vi "Address setting.vi"(7 "Address Cluster out输入":T1={"SPU"=refnum, "MPM"=[], "Port_Count"=0.0, "MPM_Count"=0.0, "SPU_Resource"=[], "USB_Resource"=[], "MPM_Communicater"="", "MPM_Count"=0.0, "MPM_Address"=[], "MPM_Portnumber"=[], "SPU_DeviveID"="", "MPM_communcation_method"=[], "TSL_sweepstartwave"=0.0, "TSL_sweepstopwave"=0.0, "TSL_Address"="", "TSL_Communicater"="", "TSL"=refnum, "tsl_communcation_method"=3, "TSL_Portnumber"=0.0} {"tsl_communcation_method" items=["GPIB", "C232C", "TCPIP", "USB"]; "MPM_communcation_method" items=["GPIB", "C232C", "TCPIP", "USB"]}, 8 "错误输入（无错误）":errorcluster caption="error in", 10 "PowerMonitorType":enum16{"DAQ", "MPM_220", "TSL_LOGG"}(ring), 11 "SPU in":refnum<k24>) -> (0 "error out":errorcluster, 1 "Address Cluster out输出":T1={"SPU"=refnum, "MPM"=[], "Port_Count"=0.0, "MPM_Count"=0.0, "SPU_Resource"=[], "USB_Resource"=[], "MPM_Communicater"="", "MPM_Count"=0.0, "MPM_Address"=[], "MPM_Portnumber"=[], "SPU_DeviveID"="", "MPM_communcation_method"=[], "TSL_sweepstartwave"=0.0, "TSL_sweepstopwave"=0.0, "TSL_Address"="", "TSL_Communicater"="", "TSL"=refnum, "tsl_communcation_method"=3, "TSL_Portnumber"=0.0} {"tsl_communcation_method" items=["GPIB", "C232C", "TCPIP", "USB"]; "MPM_communcation_method" items=["GPIB", "C232C", "TCPIP", "USB"]})   [LabVIEW 2017]
doc: "'----Apply to communication parametere from Instrument setting form"
uses:
  CTL/Address Cluster.ctl
  D:/test/ILSTS/LV_IL/LV_IL_Sample_x64/DLL/InstrumentDLL.dll
  DLL/InstrumentDLL.dll
  Share/PowerMonitorType.vi
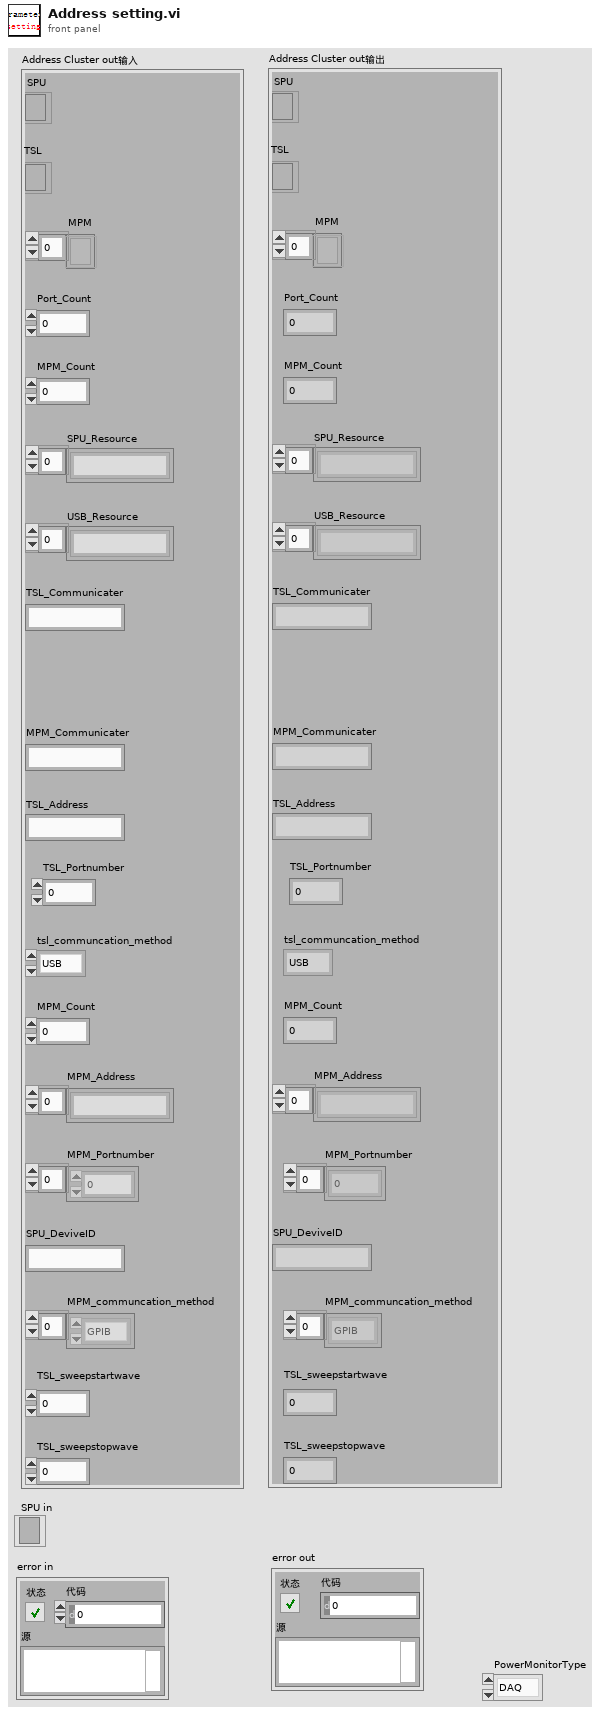
[diagram p1: front panel]
types:
  T1 = typedef "Address Cluster.ctl" = cluster{"SPU":refnum<k24>, "MPM":refnum<k24>[], "Port_Count":dbl, "MPM_Count":dbl, "SPU_Resource":string[], "USB_Resource":string[], "MPM_Communicater":string, "MPM_Count":dbl, "MPM_Address":string[], "MPM_Portnumber":dbl[], "SPU_DeviveID":string, "MPM_communcation_method":i32[], "TSL_sweepstartwave":dbl, "TSL_sweepstopwave":dbl, "TSL_Address":string, "TSL_Communicater":string, "TSL":refnum<k24>, "tsl_communcation_method":i32, "TSL_Portnumber":dbl}
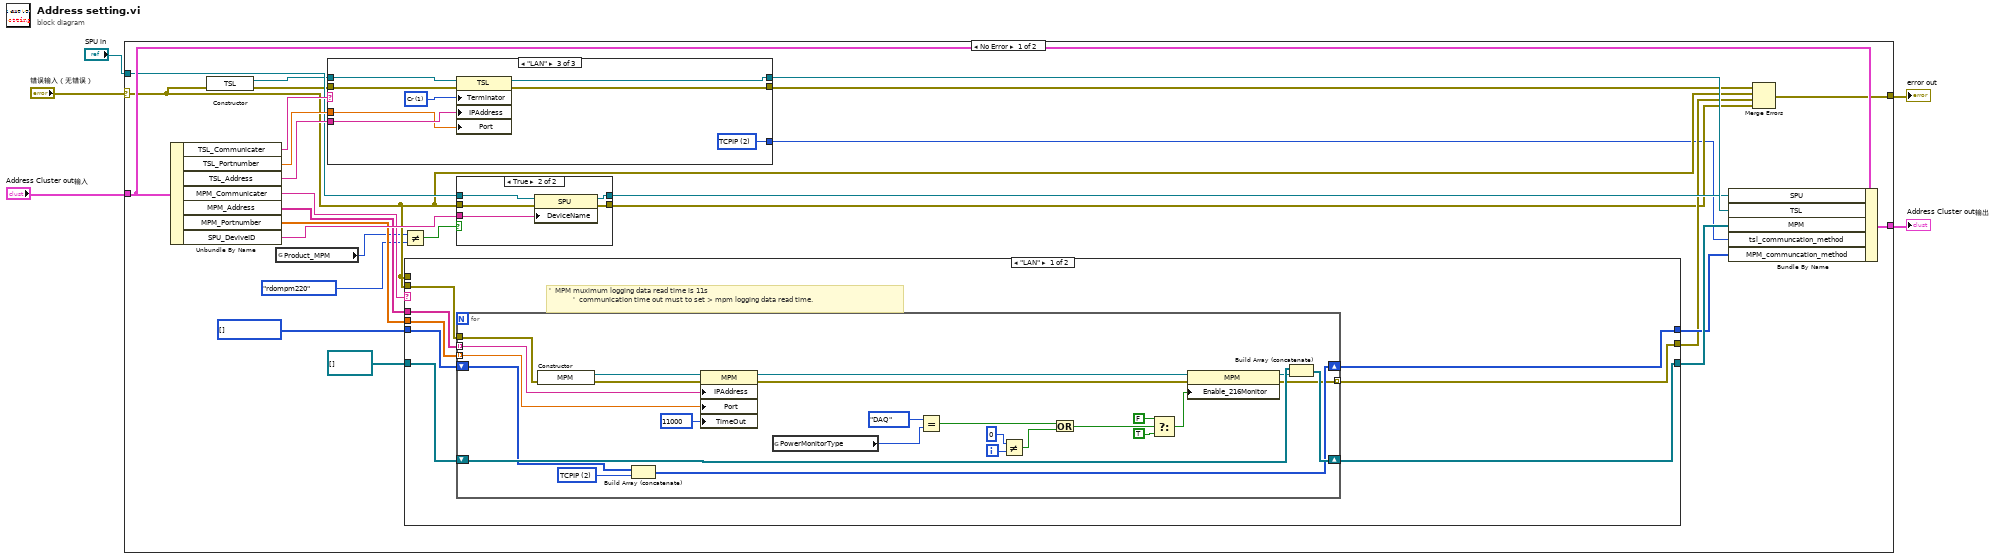
[diagram p0: block diagram]
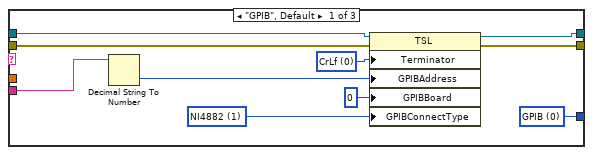
[diagram p3: hidden frame]
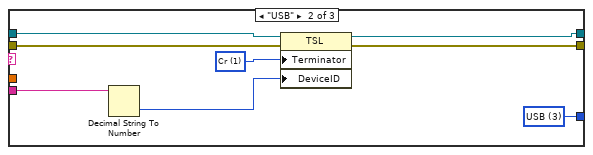
[diagram p4: hidden frame]
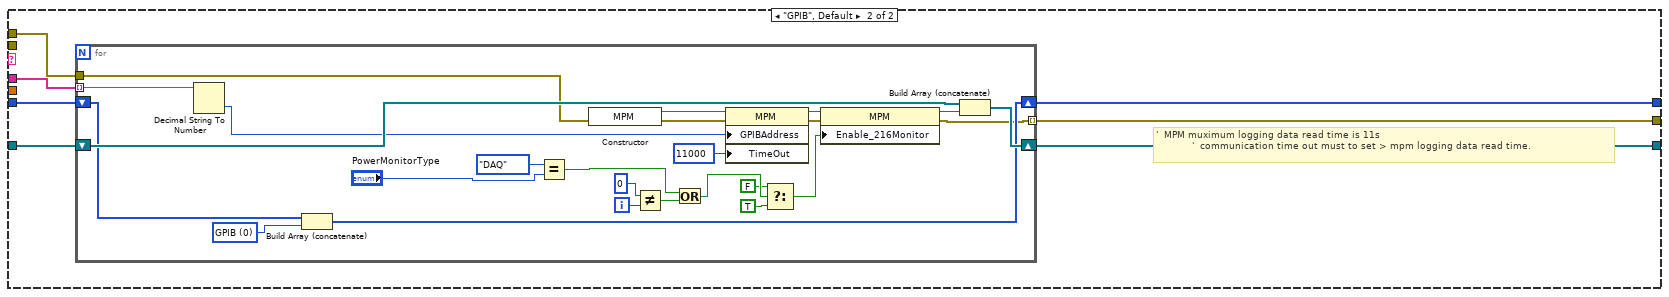
[diagram p5: hidden frame]
diagram:
  n1 = case shown="No Error" "错误输入（无错误）" {
    selector: "错误输入（无错误）" -> [w12 w132]
    tunnel: [w32 w131] -> w5
    tunnel: "Address Cluster out输入" -> [w28 w131]
    tunnel: [w14 w132] -> w3
    tunnel: "SPU in" -> [w13 _]
    frame No Error {
      w26 = i32[] [] items=["GPIB", "C232C", "TCPIP", "USB"] ("tsl_communcation_method")
      n2 = Unbundle By Name(w28) -> ("TSL_Communicater"=w19:string, "TSL_Portnumber"=w21:dbl, "TSL_Address"=w20:string, "MPM_Communicater"=w22:string, "MPM_Address"=w23:string[], "MPM_Portnumber"=w24:dbl[], "SPU_DeviveID"=w27:string)
      n3 = constructor class="TSL"(error in=w12) -> (reference out=w11:refnum<k24>, error out=w10:errorcluster)  [unwired: 2 in, 1 out]
      n4 = global read "PowerMonitorType.vi" "Product_MPM"() -> (w7:enum32{"rdompm210", "rdompm220"})
      n5 = case shown="\"LAN\"" w19 {
        tunnel: w11 -> [w49 w57 w65]
        tunnel: [w40 w50 w58] -> w31
        tunnel: w20 -> [w47 w55 w63]
        tunnel: w21 -> [_ _ w62]
        tunnel: w10 -> [w43 w53 w61]
        tunnel: [w42 w52 w60] -> w17
        tunnel: [w41 w51 w59] -> w9
        frame "GPIB", Default {
          w44 = 1 items=["NIVisa", "NI4882", "KeysightIO"] ("GPIBConnectType")
          w48 = 0 items=["CrLf", "Cr", "Lf"] ("Terminator")
          w41 = 0 items=["GPIB", "C232C", "TCPIP", "USB"] ("method")
          n6 = Decimal String To Number(string=w47) -> (number=w46:i32)  [unwired: 2 in, 1 out]
          n7 = property on="属性节点" class="TSL"(reference=w49, error in=w43, "Terminator"=w48, "GPIBAddress"=w46, "GPIBBoard"=0, "GPIBConnectType"=w44) -> (reference out=w40:refnum<k24>, error out=w42:errorcluster)
        }
        frame "USB" {
          w56 = 1 items=["CrLf", "Cr", "Lf"] ("Terminator")
          w51 = 3 items=["GPIB", "C232C", "TCPIP", "USB"] ("method")
          n8 = Decimal String To Number(string=w55) -> (number=w54:i32)  [unwired: 2 in, 1 out]
          n9 = property on="属性节点" class="TSL"(reference=w57, error in=w53, "Terminator"=w56, "DeviceID"=w54) -> (reference out=w50:refnum<k24>, error out=w52:errorcluster)
        }
        frame "LAN" {
          w64 = 1 items=["CrLf", "Cr", "Lf"] ("Terminator")
          w59 = 2 items=["GPIB", "C232C", "TCPIP", "USB"] ("method")
          n10 = property on="属性节点" class="TSL"(reference=w65, error in=w61, "Terminator"=w64, "IPAddress"=w63, "Port"=w62) -> (reference out=w58:refnum<k24>, error out=w60:errorcluster)
        }
      }
      n11 = Not Equal?(x=w7, y=enum32{"rdompm210", "rdompm220"}."rdompm220") -> (x != y?=w8:bool)
      n12 = case shown="\"LAN\"" w22 {
        tunnel: w23 -> [w73 w105]
        tunnel: w24 -> [w72 _]
        tunnel: refnum<k24>[] [] ("添加的数组") -> [w71 w104]
        tunnel: w26 -> [w70 w103]
        tunnel: [w69 w102] -> w30
        tunnel: [w68 w101] -> w18
        tunnel: [w67 w100] -> w16
        tunnel: w12 -> [_ w99]
        tunnel: w12 -> [w66 _]
        frame "LAN" {
          # "'  MPM muximum logging data read time is 11s\n            '  communication time out must to set > mpm logging data read time."
          n13 = for {
            shift-right: [w95] -> w69
            shift-left: w71 -> [w96]
            tunnel: w73 -> [w98] mode=indexing
            tunnel: w72 -> [w97] mode=indexing
            shift-right: [w92] -> w68
            shift-left: w70 -> [w94]
            tunnel: [w77] -> w67 mode=indexing
            tunnel: w66 -> [w90]
            i -> [w81]
            w93 = 2 items=["GPIB", "C232C", "TCPIP", "USB"] ("method")
            n14 = constructor class="MPM"(error in=w90) -> (reference out=w89:refnum<k24>, error out=w88:errorcluster)  [unwired: 2 in, 1 out]
            n15 = Build Array (concatenate)(w94, w93) -> (w92:i32[])
            n16 = property on="属性节点" class="MPM"(reference=w89, error in=w88, "IPAddress"=w98, "Port"=w97, "TimeOut"=11000) -> (reference out=w80:refnum<k24>, error out=w79:errorcluster)
            n17 = global read "PowerMonitorType.vi" "PowerMonitorType"() -> (w74:enum16{"DAQ", "MPM_220", "TSL_LOGG"})
            n18 = Equal?(x=enum16{"DAQ", "MPM_220", "TSL_LOGG"}."DAQ", y=w74) -> (x = y?=w83:bool)
            n19 = Not Equal?(x=0, y=w81) -> (x != y?=w82:bool)
            n20 = Or(x=w83, y=w82) -> (x .or. y?=w84:bool)
            n21 = Select(t=FALSE, s=w84, f=TRUE) -> (s? t:f=w78:bool)
            n22 = property on="属性节点" class="MPM"(reference=w80, error in=w79, "Enable_216Monitor"=w78) -> (reference out=w76:refnum<k24>, error out=w77:errorcluster)
            n23 = Build Array (concatenate)(w96, w76) -> (w95:refnum<k24>[])
          }
        }
        frame "GPIB", Default {
          # "'  MPM muximum logging data read time is 11s\n            '  communication time out must to set > mpm logging data read time."
          n24 = for {
            shift-right: [w129] -> w102
            shift-left: w104 -> [w130]
            tunnel: w105 -> [w125] mode=indexing
            shift-right: [w126] -> w101
            shift-left: w103 -> [w128]
            tunnel: [w108] -> w100 mode=indexing
            tunnel: w99 -> [w120]
            i -> [w116]
            w127 = 0 items=["GPIB", "C232C", "TCPIP", "USB"] ("method")
            n25 = Decimal String To Number(string=w125) -> (number=w123:i32)  [unwired: 2 in, 1 out]
            n26 = Build Array (concatenate)(w128, w127) -> (w126:i32[])
            n27 = Equal?(x=enum16{"DAQ", "MPM_220", "TSL_LOGG"}."DAQ", y="PowerMonitorType") -> (x = y?=w111:bool)
            n28 = constructor class="MPM"(error in=w120) -> (reference out=w122:refnum<k24>, error out=w121:errorcluster)  [unwired: 2 in, 1 out]
            n29 = Not Equal?(x=0, y=w116) -> (x != y?=w110:bool)
            n30 = Or(x=w111, y=w110) -> (x .or. y?=w112:bool)
            n31 = property on="属性节点" class="MPM"(reference=w122, error in=w121, "GPIBAddress"=w123, "TimeOut"=11000) -> (reference out=w115:refnum<k24>, error out=w114:errorcluster)
            n32 = Select(t=FALSE, s=w112, f=TRUE) -> (s? t:f=w109:bool)
            n33 = property on="属性节点" class="MPM"(reference=w115, error in=w114, "Enable_216Monitor"=w109) -> (reference out=w107:refnum<k24>, error out=w108:errorcluster)
            n34 = Build Array (concatenate)(w130, w107) -> (w129:refnum<k24>[])
          }
        }
      }
      n35 = case shown="True" w8 {
        tunnel: [w33 w39] -> w29
        tunnel: w27 -> [_ w38]
        tunnel: [w34 w37] -> w15
        tunnel: w13 -> [w33 w36]
        tunnel: w12 -> [w34 w35]
        frame False {
        }
        frame True {
          n36 = property on="属性节点" class="SPU"(reference=w36, error in=w35, "DeviceName"=w38) -> (reference out=w39:refnum<k24>, error out=w37:errorcluster)
        }
      }
      n37 = Bundle By Name(cluster=w28, "SPU"=w29, "TSL"=w31, "MPM"=w30, "tsl_communcation_method"=w9, "MPM_communcation_method"=w18) -> (w32:T1)
      n38 = Merge Errors(w17, w12, w16, w15) -> (w14:errorcluster)
    }
    frame Error {
    }
  }
  "Address Cluster out输出" <- w5
  "error out" <- w3
